vi "OCR Player Money ROI Only.vi"(7 "error in":errorcluster) -> (17 "String (Player10 Money)":string, 18 "String (Player 9 Money)":string, 19 "String (Player8 Money)":string, 20 "String (Player1 Money)":string, 21 "String (Player2 Money)":string, 22 "String (Player3 Money)":string, 23 "String (Player4 Money)":string, 24 "String (Player5 Money)":string, 25 "String (Player6 Money)":string, 26 "String (Player7 Money)":string, 27 "error out":errorcluster)   [LabVIEW 2015]
uses:
  <vilib>/vision/NI_Vision_Development_Module.lvlib
panel:
  out "appended array 2":T1(array[cluster])=[{"Global Rectangle"=[1068, 495, 1179, 512], "Contours"=[{"ID"=enum."External", "Type"=3, "Coordinates"=[1068, 495, 1179, 512]}]}, {"Global Rectangle"=[1068, 495, 1179, 512], "Contours"=[{"ID"=enum."External", "Type"=3, "Coordinates"=[1068, 495, 1179, 512]}]}, {"Global Rectangle"=[1385, 697, 1502, 712], "Contours"=[{"ID"=enum."External", "Type"=3, "Coordinates"=[1385, 697, 1502, 712]}]}, {"Global Rectangle"=[1264, 838, 1374, 853], "Contours"=[{"ID"=enum."External", "Type"=3, "Coordinates"=[1264, 838, 1374, 853]}]}, {"Global Rectangle"=[1029, 868, 1143, 884], "Contours"=[{"ID"=enum."External", "Type"=3, "Coordinates"=[1029, 868, 1143, 884]}]}, {"Global Rectangle"=[757, 870, 877, 885], "Contours"=[{"ID"=enum."External", "Type"=3, "Coordinates"=[757, 870, 877, 885]}]}, {"Global Rectangle"=[543, 836, 661, 852], "Contours"=[{"ID"=enum."External", "Type"=3, "Coordinates"=[543, 836, 661, 852]}]}, {"Global Rectangle"=[386, 689, 502, 706], "Contours"=[{"ID"=enum."External", "Type"=3, "Coordinates"=[386, 689, 502, 706]}]}, {"Global Rectangle"=[523, 533, 645, 550], "Contours"=[{"ID"=enum."External", "Type"=3, "Coordinates"=[523, 533, 645, 550]}]}, {"Global Rectangle"=[720, 494, 833, 510], "Contours"=[{"ID"=enum."External", "Type"=3, "Coordinates"=[720, 494, 833, 510]}]}]
  out "appended array":T1(array[cluster])
  out "Player Money":string[](array[string])
  in  "SS Path":path=path "c:/PokerSS/SS.png"
  out "Image Out":T2(plugin-control)
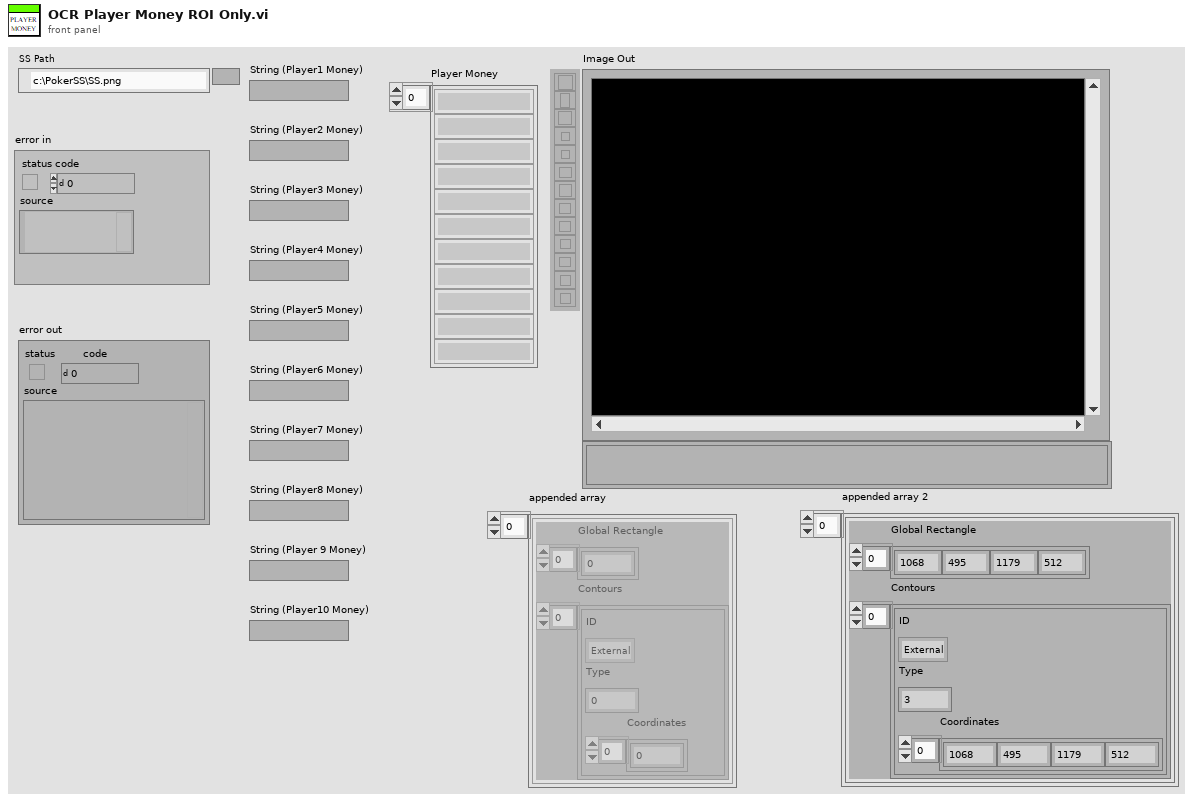
[diagram p1: front panel]
types:
  T1 = cluster{"Global Rectangle":i32[], "Contours":cluster{"ID":enum32{"External", "Internal"}, "Type":u32, "Coordinates":i32[]}[]}[]
  T2 = typedef "IMAQ Image.ctl" = refnum<image>
  T3 = cluster{"Threshold Data":cluster{"Method":enum16{"Fixed Range", "Uniform", "Linear", "Non Linear", "Local", "Color"}, "Looking for":u32, "Color Mode":u32, "Kernel Size":cluster{"Width":i32, "Height":i32}, "Ranges":cluster{"Min":i32, "Max":i32}[]}, "Reject Border":bool, "Number Of Erosions":i32, "Size & Spacing":cluster{"Segment Algorithm":u16, "Min Bounding Rect Width":i32, "Max Bounding Rect Width":i32, "Min Bounding Rect Height":i32, "Max Bounding Rect Height":i32, "Min Character Size":i32, "Max Character Size":i32, "Min Char Spacing":i32, "Max Horiz Element Spacing":i32, "Max Vert Element Spacing":i32, "Max Space Distance":i32}, "Read Options":cluster{"Read Strategy":i32, "Read Resolution":i32, "Scale Dependant":bool, "Aspect Ratio":i32, "Acceptance Level":i32, "Substitution Character":string, "MultiLine":bool}, "Valid Characters":cluster{"Pre-defined characters":i32, "User-defined characters":string}[], "Use Text Pattern":bool, "Orientation":u32, "# Lines Expected":u32, "Number of Blocks":i32}
  T4 = cluster{"Global Rectangle":i32[], "Contours":cluster{"ID":enum32{"External", "Internal"}, "Type":u32, "Coordinates":i32[]}[]}
  T5 = typedef "Image Type" = u32
  T6 = typedef "IMAQ OCR Session.ctl" = refnum<k1>
diagram:
  (unwired) path "C:/Users/Bob Dabalina/Documents/Labview/OCR Practice/Views Numbers.abc" ("File Path")
  w47 = u32 0 items=["Grayscale", "Binary", "Gradient", "Rainbow", "Temperature", "User Defined", "Binary 16 Bit", "Gradient 16 Bit", "Rainbow 16 Bit", "Temperature 16 Bit", "User Defined 16 Bit"] ("Palette Type")
  w56 = T3 {"Threshold Data"={"Method"=enum."Uniform", "Looking for"=1, "Color Mode"=0, "Kernel Size"={"Width"=32, "Height"=32}, "Ranges"=[{"Min"=1, "Max"=255}]}, "Reject Border"=TRUE, "Number Of Erosions"=0, "Size & Spacing"={"Segment Algorithm"=0, "Min Bounding Rect Width"=2, "Max Bounding Rect Width"=8, "Min Bounding Rect Height"=2, "Max Bounding Rect Height"=65536, "Min Character Size"=4, "Max Character Size"=5555, "Min Char Spacing"=1, "Max Horiz Element Spacing"=1, "Max Vert Element Spacing"=0, "Max Space Distance"=65536}, "Read Options"={"Read Strategy"=1, "Read Resolution"=2, "Scale Dependant"=FALSE, "Aspect Ratio"=400, "Acceptance Level"=700, "Substitution Character"="?", "MultiLine"=FALSE}, "Valid Characters"=[], "Use Text Pattern"=FALSE, "Orientation"=0, "# Lines Expected"=0, "Number of Blocks"=4}  # Parameters
  w2 = T4 {"Global Rectangle"=[720, 494, 833, 510], "Contours"=[{"ID"=enum."External", "Type"=3, "Coordinates"=[720, 494, 833, 510]}]}  # ROI Descriptor
  w64 = T3 {"Threshold Data"={"Method"=enum."Uniform", "Looking for"=1, "Color Mode"=0, "Kernel Size"={"Width"=32, "Height"=32}, "Ranges"=[{"Min"=1, "Max"=255}]}, "Reject Border"=TRUE, "Number Of Erosions"=0, "Size & Spacing"={"Segment Algorithm"=0, "Min Bounding Rect Width"=2, "Max Bounding Rect Width"=8, "Min Bounding Rect Height"=2, "Max Bounding Rect Height"=65536, "Min Character Size"=4, "Max Character Size"=5555, "Min Char Spacing"=1, "Max Horiz Element Spacing"=1, "Max Vert Element Spacing"=0, "Max Space Distance"=65536}, "Read Options"={"Read Strategy"=1, "Read Resolution"=2, "Scale Dependant"=FALSE, "Aspect Ratio"=400, "Acceptance Level"=700, "Substitution Character"="?", "MultiLine"=FALSE}, "Valid Characters"=[], "Use Text Pattern"=FALSE, "Orientation"=0, "# Lines Expected"=0, "Number of Blocks"=4}  # Parameters
  w4 = T4 {"Global Rectangle"=[523, 533, 645, 550], "Contours"=[{"ID"=enum."External", "Type"=3, "Coordinates"=[523, 533, 645, 550]}]}  # ROI Descriptor
  w72 = T3 {"Threshold Data"={"Method"=enum."Uniform", "Looking for"=1, "Color Mode"=0, "Kernel Size"={"Width"=32, "Height"=32}, "Ranges"=[{"Min"=1, "Max"=255}]}, "Reject Border"=TRUE, "Number Of Erosions"=0, "Size & Spacing"={"Segment Algorithm"=0, "Min Bounding Rect Width"=2, "Max Bounding Rect Width"=8, "Min Bounding Rect Height"=2, "Max Bounding Rect Height"=65536, "Min Character Size"=4, "Max Character Size"=5555, "Min Char Spacing"=1, "Max Horiz Element Spacing"=1, "Max Vert Element Spacing"=0, "Max Space Distance"=65536}, "Read Options"={"Read Strategy"=1, "Read Resolution"=2, "Scale Dependant"=FALSE, "Aspect Ratio"=400, "Acceptance Level"=700, "Substitution Character"="?", "MultiLine"=FALSE}, "Valid Characters"=[], "Use Text Pattern"=FALSE, "Orientation"=0, "# Lines Expected"=0, "Number of Blocks"=4}  # Parameters
  w6 = T4 {"Global Rectangle"=[386, 689, 502, 706], "Contours"=[{"ID"=enum."External", "Type"=3, "Coordinates"=[386, 689, 502, 706]}]}  # ROI Descriptor
  w80 = T3 {"Threshold Data"={"Method"=enum."Uniform", "Looking for"=1, "Color Mode"=0, "Kernel Size"={"Width"=32, "Height"=32}, "Ranges"=[{"Min"=1, "Max"=255}]}, "Reject Border"=TRUE, "Number Of Erosions"=0, "Size & Spacing"={"Segment Algorithm"=0, "Min Bounding Rect Width"=2, "Max Bounding Rect Width"=8, "Min Bounding Rect Height"=2, "Max Bounding Rect Height"=65536, "Min Character Size"=4, "Max Character Size"=5555, "Min Char Spacing"=1, "Max Horiz Element Spacing"=1, "Max Vert Element Spacing"=0, "Max Space Distance"=65536}, "Read Options"={"Read Strategy"=1, "Read Resolution"=2, "Scale Dependant"=FALSE, "Aspect Ratio"=400, "Acceptance Level"=700, "Substitution Character"="?", "MultiLine"=FALSE}, "Valid Characters"=[], "Use Text Pattern"=FALSE, "Orientation"=0, "# Lines Expected"=0, "Number of Blocks"=4}  # Parameters
  w8 = T4 {"Global Rectangle"=[543, 836, 661, 852], "Contours"=[{"ID"=enum."External", "Type"=3, "Coordinates"=[543, 836, 661, 852]}]}  # ROI Descriptor
  w88 = T3 {"Threshold Data"={"Method"=enum."Uniform", "Looking for"=1, "Color Mode"=0, "Kernel Size"={"Width"=32, "Height"=32}, "Ranges"=[{"Min"=1, "Max"=255}]}, "Reject Border"=TRUE, "Number Of Erosions"=0, "Size & Spacing"={"Segment Algorithm"=0, "Min Bounding Rect Width"=2, "Max Bounding Rect Width"=8, "Min Bounding Rect Height"=2, "Max Bounding Rect Height"=65536, "Min Character Size"=4, "Max Character Size"=5555, "Min Char Spacing"=1, "Max Horiz Element Spacing"=1, "Max Vert Element Spacing"=0, "Max Space Distance"=65536}, "Read Options"={"Read Strategy"=1, "Read Resolution"=2, "Scale Dependant"=FALSE, "Aspect Ratio"=400, "Acceptance Level"=700, "Substitution Character"="?", "MultiLine"=FALSE}, "Valid Characters"=[], "Use Text Pattern"=FALSE, "Orientation"=0, "# Lines Expected"=0, "Number of Blocks"=4}  # Parameters
  w10 = T4 {"Global Rectangle"=[757, 870, 877, 885], "Contours"=[{"ID"=enum."External", "Type"=3, "Coordinates"=[757, 870, 877, 885]}]}  # ROI Descriptor
  w96 = T3 {"Threshold Data"={"Method"=enum."Uniform", "Looking for"=1, "Color Mode"=0, "Kernel Size"={"Width"=32, "Height"=32}, "Ranges"=[{"Min"=1, "Max"=255}]}, "Reject Border"=TRUE, "Number Of Erosions"=0, "Size & Spacing"={"Segment Algorithm"=0, "Min Bounding Rect Width"=2, "Max Bounding Rect Width"=8, "Min Bounding Rect Height"=2, "Max Bounding Rect Height"=65536, "Min Character Size"=4, "Max Character Size"=5555, "Min Char Spacing"=1, "Max Horiz Element Spacing"=1, "Max Vert Element Spacing"=0, "Max Space Distance"=65536}, "Read Options"={"Read Strategy"=1, "Read Resolution"=2, "Scale Dependant"=FALSE, "Aspect Ratio"=400, "Acceptance Level"=700, "Substitution Character"="?", "MultiLine"=FALSE}, "Valid Characters"=[], "Use Text Pattern"=FALSE, "Orientation"=0, "# Lines Expected"=0, "Number of Blocks"=4}  # Parameters
  w12 = T4 {"Global Rectangle"=[1029, 868, 1143, 884], "Contours"=[{"ID"=enum."External", "Type"=3, "Coordinates"=[1029, 868, 1143, 884]}]}  # ROI Descriptor
  w104 = T3 {"Threshold Data"={"Method"=enum."Uniform", "Looking for"=1, "Color Mode"=0, "Kernel Size"={"Width"=32, "Height"=32}, "Ranges"=[{"Min"=1, "Max"=255}]}, "Reject Border"=TRUE, "Number Of Erosions"=0, "Size & Spacing"={"Segment Algorithm"=0, "Min Bounding Rect Width"=2, "Max Bounding Rect Width"=8, "Min Bounding Rect Height"=2, "Max Bounding Rect Height"=65536, "Min Character Size"=4, "Max Character Size"=5555, "Min Char Spacing"=1, "Max Horiz Element Spacing"=1, "Max Vert Element Spacing"=0, "Max Space Distance"=65536}, "Read Options"={"Read Strategy"=1, "Read Resolution"=2, "Scale Dependant"=FALSE, "Aspect Ratio"=400, "Acceptance Level"=700, "Substitution Character"="?", "MultiLine"=FALSE}, "Valid Characters"=[], "Use Text Pattern"=FALSE, "Orientation"=0, "# Lines Expected"=0, "Number of Blocks"=4}  # Parameters
  w14 = T4 {"Global Rectangle"=[1264, 838, 1374, 853], "Contours"=[{"ID"=enum."External", "Type"=3, "Coordinates"=[1264, 838, 1374, 853]}]}  # ROI Descriptor
  w112 = T3 {"Threshold Data"={"Method"=enum."Uniform", "Looking for"=1, "Color Mode"=0, "Kernel Size"={"Width"=32, "Height"=32}, "Ranges"=[{"Min"=1, "Max"=255}]}, "Reject Border"=TRUE, "Number Of Erosions"=0, "Size & Spacing"={"Segment Algorithm"=0, "Min Bounding Rect Width"=2, "Max Bounding Rect Width"=8, "Min Bounding Rect Height"=2, "Max Bounding Rect Height"=65536, "Min Character Size"=4, "Max Character Size"=5555, "Min Char Spacing"=1, "Max Horiz Element Spacing"=1, "Max Vert Element Spacing"=0, "Max Space Distance"=65536}, "Read Options"={"Read Strategy"=1, "Read Resolution"=2, "Scale Dependant"=FALSE, "Aspect Ratio"=400, "Acceptance Level"=700, "Substitution Character"="?", "MultiLine"=FALSE}, "Valid Characters"=[], "Use Text Pattern"=FALSE, "Orientation"=0, "# Lines Expected"=0, "Number of Blocks"=4}  # Parameters
  w16 = T4 {"Global Rectangle"=[1385, 697, 1502, 712], "Contours"=[{"ID"=enum."External", "Type"=3, "Coordinates"=[1385, 697, 1502, 712]}]}  # ROI Descriptor
  w120 = T3 {"Threshold Data"={"Method"=enum."Uniform", "Looking for"=1, "Color Mode"=0, "Kernel Size"={"Width"=32, "Height"=32}, "Ranges"=[{"Min"=1, "Max"=255}]}, "Reject Border"=TRUE, "Number Of Erosions"=0, "Size & Spacing"={"Segment Algorithm"=0, "Min Bounding Rect Width"=2, "Max Bounding Rect Width"=8, "Min Bounding Rect Height"=2, "Max Bounding Rect Height"=65536, "Min Character Size"=4, "Max Character Size"=5555, "Min Char Spacing"=1, "Max Horiz Element Spacing"=1, "Max Vert Element Spacing"=0, "Max Space Distance"=65536}, "Read Options"={"Read Strategy"=1, "Read Resolution"=2, "Scale Dependant"=FALSE, "Aspect Ratio"=400, "Acceptance Level"=700, "Substitution Character"="?", "MultiLine"=FALSE}, "Valid Characters"=[], "Use Text Pattern"=FALSE, "Orientation"=0, "# Lines Expected"=0, "Number of Blocks"=4}  # Parameters
  w18 = T4 {"Global Rectangle"=[1068, 495, 1179, 512], "Contours"=[{"ID"=enum."External", "Type"=3, "Coordinates"=[1068, 495, 1179, 512]}]}  # ROI Descriptor
  w128 = T3 {"Threshold Data"={"Method"=enum."Uniform", "Looking for"=1, "Color Mode"=0, "Kernel Size"={"Width"=32, "Height"=32}, "Ranges"=[{"Min"=1, "Max"=255}]}, "Reject Border"=TRUE, "Number Of Erosions"=0, "Size & Spacing"={"Segment Algorithm"=0, "Min Bounding Rect Width"=2, "Max Bounding Rect Width"=8, "Min Bounding Rect Height"=2, "Max Bounding Rect Height"=65536, "Min Character Size"=4, "Max Character Size"=5555, "Min Char Spacing"=1, "Max Horiz Element Spacing"=1, "Max Vert Element Spacing"=0, "Max Space Distance"=65536}, "Read Options"={"Read Strategy"=1, "Read Resolution"=2, "Scale Dependant"=FALSE, "Aspect Ratio"=400, "Acceptance Level"=700, "Substitution Character"="?", "MultiLine"=FALSE}, "Valid Characters"=[], "Use Text Pattern"=FALSE, "Orientation"=0, "# Lines Expected"=0, "Number of Blocks"=4}  # Parameters
  w21 = T4 {"Global Rectangle"=[1068, 495, 1179, 512], "Contours"=[{"ID"=enum."External", "Type"=3, "Coordinates"=[1068, 495, 1179, 512]}]}  # ROI Descriptor
  w131 = 1 items=["Red", "Green", "Blue", "Hue", "Saturation", "Luminance", "Value", "Intensity"] ("Color Plane")
  w132 = T5 4 items=["Grayscale (U8)", "Grayscale (I16)", "Grayscale (SGL)", "Complex (CSG)", "RGB (U32)", "HSL (U32)", "RGB (U64)", "Grayscale (U16)"] ("Image Type")
  # "Create player money array"
  n1 = Call Chain() -> (call chain=w134:string[])
  n2 = Index Array(array=w134) -> (element=w133:string)  [unwired: 1 in]
  n3 = call "IMAQ Create"("Image Name"=w133, "Image Type"=w132, "error in (no error)"="error in") -> ("New Image"=w137:T2, "error out"=w136:errorcluster)  [unwired: 1 in, 1 out]
  n4 = call "IMAQ ReadFile"("File Path"="SS Path", "error in (no error)"=w136, "Image"=w137) -> ("error out"=w138:errorcluster, "Image Out"=w130:T2)  [unwired: 2 in, 5 out]
  n5 = call "IMAQ ExtractSingleColorPlane"("Color Plane"=w131, "error in (no error)"=w138, "Image Src"=w130) -> ("error out"=w129:errorcluster, "Image Dst Out"=w48:T2)  [unwired: 1 in, 6 out]
  "Image Out" <- w48
  n6 = Initialize Array(w21, 1 ("dimension size")) -> (w19:T1)
  n7 = while "Create an OCR session and read the character set file.\nSet paramaters from Vision Assistant Step." {
    shift-right: [w143] -> w126
    shift-left: _ -> [w142]
    tunnel: w129 -> [w145]
    tunnel: w128 -> [w141]
    tunnel: path "C:/Users/Bob Dabalina/Documents/Labview/OCR Practice/Views Numbers.abc" ("File Path") -> [w140]
    tunnel: [w139] -> w127
    stop <- FALSE continue-if-true
    n8 = First Call?() -> (First Call?: T/F=w144:bool)
    n9 = case shown="True" w144 {
      tunnel: w140 -> [_ w152]
      tunnel: w145 -> [w147 w156]
      tunnel: [w148 w154] -> w143
      tunnel: [w147 w153] -> w139
      tunnel: w141 -> [_ w149]
      tunnel: w142 -> [w148 _]
      frame False {
      }
      frame True {
        w157 = 0 items=["Read All", "Read Character Set Only", "Read Properties Only"] ("Read Options")
        n10 = call <vilib>:"IVA Get Alternate Path.vi"("Path In"=w152) -> ("Path Out"=w151:path)  [unwired: 10 out]
        n11 = call "IMAQ OCR Create Session"("error in (no error)"=w156) -> ("error out"=w158:errorcluster, "IMAQ OCR Session"=w159:T6)  [unwired: 9 out]
        n12 = call "IMAQ OCR Read Character Set File"("File Path"=w151, "error in (no error)"=w158, "Read Options"=w157, "IMAQ OCR Session"=w159) -> ("error out"=w155:errorcluster, "IMAQ OCR Session (dup)"=w150:T6)  [unwired: 1 in, 5 out]
        n13 = call <vilib>:"IVA OCR - Set Parameters 2.vi"("error in (no error)"=w155, "Parameters"=w149, "IMAQ OCR Session"=w150) -> ("error out"=w153:errorcluster, "IMAQ OCR Session Out"=w154:T6)  [unwired: 7 in]
      }
    }
  }
  n14 = Unbundle By Name(w128) -> ("# Lines Expected"=w124:u32, "Orientation"=w125:u32)
  n15 = call "IMAQ OCR Read Text 4"("IMAQ OCR Session"=w126, "ROI Descriptor"=w21, "Image"=w48, "Number of Lines Requested"=w124, "error in (no error)"=w127, "Orientation"=w125) -> ("Read String"=w41:string, "error out"=w123:errorcluster)  [unwired: 8 out]
  "String (Player1 Money)" <- w41
  n16 = call <vilib>:"IVA Clear Coordsys Errors.vi"("error in (no error)"=w123) -> ("error out"=w122:errorcluster)  [unwired: 10 in]
  n17 = Initialize Array("") -> (w43:string[])  [unwired: 1 in]
  n18 = Insert Into Array(array=w43, index=0, new element=w41) -> (w40:string[])
  n19 = Build Array (concatenate)(w19, w18) -> (w17:T1)
  n20 = while "Create an OCR session and read the character set file.\nSet paramaters from Vision Assistant Step." {
    shift-right: [w164] -> w118
    shift-left: _ -> [w163]
    tunnel: w122 -> [w166]
    tunnel: w120 -> [w162]
    tunnel: path "C:/Users/Bob Dabalina/Documents/Labview/OCR Practice/Views Numbers.abc" ("File Path") -> [w161]
    tunnel: [w160] -> w119
    stop <- FALSE continue-if-true
    n21 = First Call?() -> (First Call?: T/F=w165:bool)
    n22 = case shown="True" w165 {
      tunnel: w161 -> [_ w173]
      tunnel: w166 -> [w168 w177]
      tunnel: [w169 w175] -> w164
      tunnel: [w168 w174] -> w160
      tunnel: w162 -> [_ w170]
      tunnel: w163 -> [w169 _]
      frame False {
      }
      frame True {
        w178 = 0 items=["Read All", "Read Character Set Only", "Read Properties Only"] ("Read Options")
        n23 = call <vilib>:"IVA Get Alternate Path.vi"("Path In"=w173) -> ("Path Out"=w172:path)  [unwired: 10 out]
        n24 = call "IMAQ OCR Create Session"("error in (no error)"=w177) -> ("error out"=w179:errorcluster, "IMAQ OCR Session"=w180:T6)  [unwired: 9 out]
        n25 = call "IMAQ OCR Read Character Set File"("File Path"=w172, "error in (no error)"=w179, "Read Options"=w178, "IMAQ OCR Session"=w180) -> ("error out"=w176:errorcluster, "IMAQ OCR Session (dup)"=w171:T6)  [unwired: 1 in, 5 out]
        n26 = call <vilib>:"IVA OCR - Set Parameters 2.vi"("error in (no error)"=w176, "Parameters"=w170, "IMAQ OCR Session"=w171) -> ("error out"=w174:errorcluster, "IMAQ OCR Session Out"=w175:T6)  [unwired: 7 in]
      }
    }
  }
  n27 = Unbundle By Name(w120) -> ("# Lines Expected"=w116:u32, "Orientation"=w117:u32)
  n28 = call "IMAQ OCR Read Text 4"("IMAQ OCR Session"=w118, "ROI Descriptor"=w18, "Image"=w48, "Number of Lines Requested"=w116, "error in (no error)"=w119, "Orientation"=w117) -> ("Read String"=w39:string, "error out"=w115:errorcluster)  [unwired: 8 out]
  "String (Player2 Money)" <- w39
  n29 = call <vilib>:"IVA Clear Coordsys Errors.vi"("error in (no error)"=w115) -> ("error out"=w114:errorcluster)  [unwired: 10 in]
  n30 = Build Array (concatenate)(w40, w39) -> (w38:string[])
  n31 = Build Array (concatenate)(w17, w16) -> (w15:T1)
  n32 = while "Create an OCR session and read the character set file.\nSet paramaters from Vision Assistant Step." {
    shift-right: [w185] -> w110
    shift-left: _ -> [w184]
    tunnel: w114 -> [w187]
    tunnel: w112 -> [w183]
    tunnel: path "C:/Users/Bob Dabalina/Documents/Labview/OCR Practice/Views Numbers.abc" ("File Path") -> [w182]
    tunnel: [w181] -> w111
    stop <- FALSE continue-if-true
    n33 = First Call?() -> (First Call?: T/F=w186:bool)
    n34 = case shown="True" w186 {
      tunnel: w182 -> [_ w194]
      tunnel: w187 -> [w189 w198]
      tunnel: [w190 w196] -> w185
      tunnel: [w189 w195] -> w181
      tunnel: w183 -> [_ w191]
      tunnel: w184 -> [w190 _]
      frame False {
      }
      frame True {
        w199 = 0 items=["Read All", "Read Character Set Only", "Read Properties Only"] ("Read Options")
        n35 = call <vilib>:"IVA Get Alternate Path.vi"("Path In"=w194) -> ("Path Out"=w193:path)  [unwired: 10 out]
        n36 = call "IMAQ OCR Create Session"("error in (no error)"=w198) -> ("error out"=w200:errorcluster, "IMAQ OCR Session"=w201:T6)  [unwired: 9 out]
        n37 = call "IMAQ OCR Read Character Set File"("File Path"=w193, "error in (no error)"=w200, "Read Options"=w199, "IMAQ OCR Session"=w201) -> ("error out"=w197:errorcluster, "IMAQ OCR Session (dup)"=w192:T6)  [unwired: 1 in, 5 out]
        n38 = call <vilib>:"IVA OCR - Set Parameters 2.vi"("error in (no error)"=w197, "Parameters"=w191, "IMAQ OCR Session"=w192) -> ("error out"=w195:errorcluster, "IMAQ OCR Session Out"=w196:T6)  [unwired: 7 in]
      }
    }
  }
  n39 = Unbundle By Name(w112) -> ("# Lines Expected"=w108:u32, "Orientation"=w109:u32)
  n40 = call "IMAQ OCR Read Text 4"("IMAQ OCR Session"=w110, "ROI Descriptor"=w16, "Image"=w48, "Number of Lines Requested"=w108, "error in (no error)"=w111, "Orientation"=w109) -> ("Read String"=w37:string, "error out"=w107:errorcluster)  [unwired: 8 out]
  "String (Player3 Money)" <- w37
  n41 = call <vilib>:"IVA Clear Coordsys Errors.vi"("error in (no error)"=w107) -> ("error out"=w106:errorcluster)  [unwired: 10 in]
  n42 = Build Array (concatenate)(w38, w37) -> (w36:string[])
  n43 = Build Array (concatenate)(w15, w14) -> (w13:T1)
  n44 = while "Create an OCR session and read the character set file.\nSet paramaters from Vision Assistant Step." {
    shift-right: [w206] -> w102
    shift-left: _ -> [w205]
    tunnel: w106 -> [w208]
    tunnel: w104 -> [w204]
    tunnel: path "C:/Users/Bob Dabalina/Documents/Labview/OCR Practice/Views Numbers.abc" ("File Path") -> [w203]
    tunnel: [w202] -> w103
    stop <- FALSE continue-if-true
    n45 = First Call?() -> (First Call?: T/F=w207:bool)
    n46 = case shown="True" w207 {
      tunnel: w203 -> [_ w215]
      tunnel: w208 -> [w210 w219]
      tunnel: [w211 w217] -> w206
      tunnel: [w210 w216] -> w202
      tunnel: w204 -> [_ w212]
      tunnel: w205 -> [w211 _]
      frame False {
      }
      frame True {
        w220 = 0 items=["Read All", "Read Character Set Only", "Read Properties Only"] ("Read Options")
        n47 = call <vilib>:"IVA Get Alternate Path.vi"("Path In"=w215) -> ("Path Out"=w214:path)  [unwired: 10 out]
        n48 = call "IMAQ OCR Create Session"("error in (no error)"=w219) -> ("error out"=w221:errorcluster, "IMAQ OCR Session"=w222:T6)  [unwired: 9 out]
        n49 = call "IMAQ OCR Read Character Set File"("File Path"=w214, "error in (no error)"=w221, "Read Options"=w220, "IMAQ OCR Session"=w222) -> ("error out"=w218:errorcluster, "IMAQ OCR Session (dup)"=w213:T6)  [unwired: 1 in, 5 out]
        n50 = call <vilib>:"IVA OCR - Set Parameters 2.vi"("error in (no error)"=w218, "Parameters"=w212, "IMAQ OCR Session"=w213) -> ("error out"=w216:errorcluster, "IMAQ OCR Session Out"=w217:T6)  [unwired: 7 in]
      }
    }
  }
  n51 = Unbundle By Name(w104) -> ("# Lines Expected"=w100:u32, "Orientation"=w101:u32)
  n52 = call "IMAQ OCR Read Text 4"("IMAQ OCR Session"=w102, "ROI Descriptor"=w14, "Image"=w48, "Number of Lines Requested"=w100, "error in (no error)"=w103, "Orientation"=w101) -> ("Read String"=w35:string, "error out"=w99:errorcluster)  [unwired: 8 out]
  "String (Player4 Money)" <- w35
  n53 = call <vilib>:"IVA Clear Coordsys Errors.vi"("error in (no error)"=w99) -> ("error out"=w98:errorcluster)  [unwired: 10 in]
  n54 = Build Array (concatenate)(w36, w35) -> (w34:string[])
  n55 = Build Array (concatenate)(w13, w12) -> (w11:T1)
  n56 = while "Create an OCR session and read the character set file.\nSet paramaters from Vision Assistant Step." {
    shift-right: [w227] -> w94
    shift-left: _ -> [w226]
    tunnel: w98 -> [w229]
    tunnel: w96 -> [w225]
    tunnel: path "C:/Users/Bob Dabalina/Documents/Labview/OCR Practice/Views Numbers.abc" ("File Path") -> [w224]
    tunnel: [w223] -> w95
    stop <- FALSE continue-if-true
    n57 = First Call?() -> (First Call?: T/F=w228:bool)
    n58 = case shown="True" w228 {
      tunnel: w224 -> [_ w236]
      tunnel: w229 -> [w231 w240]
      tunnel: [w232 w238] -> w227
      tunnel: [w231 w237] -> w223
      tunnel: w225 -> [_ w233]
      tunnel: w226 -> [w232 _]
      frame False {
      }
      frame True {
        w241 = 0 items=["Read All", "Read Character Set Only", "Read Properties Only"] ("Read Options")
        n59 = call <vilib>:"IVA Get Alternate Path.vi"("Path In"=w236) -> ("Path Out"=w235:path)  [unwired: 10 out]
        n60 = call "IMAQ OCR Create Session"("error in (no error)"=w240) -> ("error out"=w242:errorcluster, "IMAQ OCR Session"=w243:T6)  [unwired: 9 out]
        n61 = call "IMAQ OCR Read Character Set File"("File Path"=w235, "error in (no error)"=w242, "Read Options"=w241, "IMAQ OCR Session"=w243) -> ("error out"=w239:errorcluster, "IMAQ OCR Session (dup)"=w234:T6)  [unwired: 1 in, 5 out]
        n62 = call <vilib>:"IVA OCR - Set Parameters 2.vi"("error in (no error)"=w239, "Parameters"=w233, "IMAQ OCR Session"=w234) -> ("error out"=w237:errorcluster, "IMAQ OCR Session Out"=w238:T6)  [unwired: 7 in]
      }
    }
  }
  n63 = Unbundle By Name(w96) -> ("# Lines Expected"=w92:u32, "Orientation"=w93:u32)
  n64 = call "IMAQ OCR Read Text 4"("IMAQ OCR Session"=w94, "ROI Descriptor"=w12, "Image"=w48, "Number of Lines Requested"=w92, "error in (no error)"=w95, "Orientation"=w93) -> ("Read String"=w33:string, "error out"=w91:errorcluster)  [unwired: 8 out]
  "String (Player5 Money)" <- w33
  n65 = call <vilib>:"IVA Clear Coordsys Errors.vi"("error in (no error)"=w91) -> ("error out"=w90:errorcluster)  [unwired: 10 in]
  n66 = Build Array (concatenate)(w34, w33) -> (w32:string[])
  n67 = Build Array (concatenate)(w11, w10) -> (w9:T1)
  n68 = while "Create an OCR session and read the character set file.\nSet paramaters from Vision Assistant Step." {
    shift-right: [w248] -> w86
    shift-left: _ -> [w247]
    tunnel: w90 -> [w250]
    tunnel: w88 -> [w246]
    tunnel: path "C:/Users/Bob Dabalina/Documents/Labview/OCR Practice/Views Numbers.abc" ("File Path") -> [w245]
    tunnel: [w244] -> w87
    stop <- FALSE continue-if-true
    n69 = First Call?() -> (First Call?: T/F=w249:bool)
    n70 = case shown="True" w249 {
      tunnel: w245 -> [_ w257]
      tunnel: w250 -> [w252 w261]
      tunnel: [w253 w259] -> w248
      tunnel: [w252 w258] -> w244
      tunnel: w246 -> [_ w254]
      tunnel: w247 -> [w253 _]
      frame False {
      }
      frame True {
        w262 = 0 items=["Read All", "Read Character Set Only", "Read Properties Only"] ("Read Options")
        n71 = call <vilib>:"IVA Get Alternate Path.vi"("Path In"=w257) -> ("Path Out"=w256:path)  [unwired: 10 out]
        n72 = call "IMAQ OCR Create Session"("error in (no error)"=w261) -> ("error out"=w263:errorcluster, "IMAQ OCR Session"=w264:T6)  [unwired: 9 out]
        n73 = call "IMAQ OCR Read Character Set File"("File Path"=w256, "error in (no error)"=w263, "Read Options"=w262, "IMAQ OCR Session"=w264) -> ("error out"=w260:errorcluster, "IMAQ OCR Session (dup)"=w255:T6)  [unwired: 1 in, 5 out]
        n74 = call <vilib>:"IVA OCR - Set Parameters 2.vi"("error in (no error)"=w260, "Parameters"=w254, "IMAQ OCR Session"=w255) -> ("error out"=w258:errorcluster, "IMAQ OCR Session Out"=w259:T6)  [unwired: 7 in]
      }
    }
  }
  n75 = Unbundle By Name(w88) -> ("# Lines Expected"=w84:u32, "Orientation"=w85:u32)
  n76 = call "IMAQ OCR Read Text 4"("IMAQ OCR Session"=w86, "ROI Descriptor"=w10, "Image"=w48, "Number of Lines Requested"=w84, "error in (no error)"=w87, "Orientation"=w85) -> ("Read String"=w31:string, "error out"=w83:errorcluster)  [unwired: 8 out]
  "String (Player6 Money)" <- w31
  n77 = call <vilib>:"IVA Clear Coordsys Errors.vi"("error in (no error)"=w83) -> ("error out"=w82:errorcluster)  [unwired: 10 in]
  n78 = Build Array (concatenate)(w32, w31) -> (w30:string[])
  n79 = Build Array (concatenate)(w9, w8) -> (w7:T1)
  n80 = while "Create an OCR session and read the character set file.\nSet paramaters from Vision Assistant Step." {
    shift-right: [w269] -> w78
    shift-left: _ -> [w268]
    tunnel: w82 -> [w271]
    tunnel: w80 -> [w267]
    tunnel: path "C:/Users/Bob Dabalina/Documents/Labview/OCR Practice/Views Numbers.abc" ("File Path") -> [w266]
    tunnel: [w265] -> w79
    stop <- FALSE continue-if-true
    n81 = First Call?() -> (First Call?: T/F=w270:bool)
    n82 = case shown="True" w270 {
      tunnel: w266 -> [_ w278]
      tunnel: w271 -> [w273 w282]
      tunnel: [w274 w280] -> w269
      tunnel: [w273 w279] -> w265
      tunnel: w267 -> [_ w275]
      tunnel: w268 -> [w274 _]
      frame False {
      }
      frame True {
        w283 = 0 items=["Read All", "Read Character Set Only", "Read Properties Only"] ("Read Options")
        n83 = call <vilib>:"IVA Get Alternate Path.vi"("Path In"=w278) -> ("Path Out"=w277:path)  [unwired: 10 out]
        n84 = call "IMAQ OCR Create Session"("error in (no error)"=w282) -> ("error out"=w284:errorcluster, "IMAQ OCR Session"=w285:T6)  [unwired: 9 out]
        n85 = call "IMAQ OCR Read Character Set File"("File Path"=w277, "error in (no error)"=w284, "Read Options"=w283, "IMAQ OCR Session"=w285) -> ("error out"=w281:errorcluster, "IMAQ OCR Session (dup)"=w276:T6)  [unwired: 1 in, 5 out]
        n86 = call <vilib>:"IVA OCR - Set Parameters 2.vi"("error in (no error)"=w281, "Parameters"=w275, "IMAQ OCR Session"=w276) -> ("error out"=w279:errorcluster, "IMAQ OCR Session Out"=w280:T6)  [unwired: 7 in]
      }
    }
  }
  n87 = Unbundle By Name(w80) -> ("# Lines Expected"=w76:u32, "Orientation"=w77:u32)
  n88 = call "IMAQ OCR Read Text 4"("IMAQ OCR Session"=w78, "ROI Descriptor"=w8, "Image"=w48, "Number of Lines Requested"=w76, "error in (no error)"=w79, "Orientation"=w77) -> ("Read String"=w29:string, "error out"=w75:errorcluster)  [unwired: 8 out]
  "String (Player7 Money)" <- w29
  n89 = call <vilib>:"IVA Clear Coordsys Errors.vi"("error in (no error)"=w75) -> ("error out"=w74:errorcluster)  [unwired: 10 in]
  n90 = Build Array (concatenate)(w30, w29) -> (w28:string[])
  n91 = Build Array (concatenate)(w7, w6) -> (w5:T1)
  n92 = while "Create an OCR session and read the character set file.\nSet paramaters from Vision Assistant Step." {
    shift-right: [w290] -> w70
    shift-left: _ -> [w289]
    tunnel: w74 -> [w292]
    tunnel: w72 -> [w288]
    tunnel: path "C:/Users/Bob Dabalina/Documents/Labview/OCR Practice/Views Numbers.abc" ("File Path") -> [w287]
    tunnel: [w286] -> w71
    stop <- FALSE continue-if-true
    n93 = First Call?() -> (First Call?: T/F=w291:bool)
    n94 = case shown="True" w291 {
      tunnel: w287 -> [_ w299]
      tunnel: w292 -> [w294 w303]
      tunnel: [w295 w301] -> w290
      tunnel: [w294 w300] -> w286
      tunnel: w288 -> [_ w296]
      tunnel: w289 -> [w295 _]
      frame False {
      }
      frame True {
        w304 = 0 items=["Read All", "Read Character Set Only", "Read Properties Only"] ("Read Options")
        n95 = call <vilib>:"IVA Get Alternate Path.vi"("Path In"=w299) -> ("Path Out"=w298:path)  [unwired: 10 out]
        n96 = call "IMAQ OCR Create Session"("error in (no error)"=w303) -> ("error out"=w305:errorcluster, "IMAQ OCR Session"=w306:T6)  [unwired: 9 out]
        n97 = call "IMAQ OCR Read Character Set File"("File Path"=w298, "error in (no error)"=w305, "Read Options"=w304, "IMAQ OCR Session"=w306) -> ("error out"=w302:errorcluster, "IMAQ OCR Session (dup)"=w297:T6)  [unwired: 1 in, 5 out]
        n98 = call <vilib>:"IVA OCR - Set Parameters 2.vi"("error in (no error)"=w302, "Parameters"=w296, "IMAQ OCR Session"=w297) -> ("error out"=w300:errorcluster, "IMAQ OCR Session Out"=w301:T6)  [unwired: 7 in]
      }
    }
  }
  n99 = Unbundle By Name(w72) -> ("# Lines Expected"=w68:u32, "Orientation"=w69:u32)
  n100 = call "IMAQ OCR Read Text 4"("IMAQ OCR Session"=w70, "ROI Descriptor"=w6, "Image"=w48, "Number of Lines Requested"=w68, "error in (no error)"=w71, "Orientation"=w69) -> ("Read String"=w27:string, "error out"=w67:errorcluster)  [unwired: 8 out]
  "String (Player8 Money)" <- w27
  n101 = call <vilib>:"IVA Clear Coordsys Errors.vi"("error in (no error)"=w67) -> ("error out"=w66:errorcluster)  [unwired: 10 in]
  n102 = Build Array (concatenate)(w28, w27) -> (w26:string[])
  n103 = Build Array (concatenate)(w5, w4) -> (w3:T1)
  n104 = while "Create an OCR session and read the character set file.\nSet paramaters from Vision Assistant Step." {
    shift-right: [w311] -> w62
    shift-left: _ -> [w310]
    tunnel: w66 -> [w313]
    tunnel: w64 -> [w309]
    tunnel: path "C:/Users/Bob Dabalina/Documents/Labview/OCR Practice/Views Numbers.abc" ("File Path") -> [w308]
    tunnel: [w307] -> w63
    stop <- FALSE continue-if-true
    n105 = First Call?() -> (First Call?: T/F=w312:bool)
    n106 = case shown="True" w312 {
      tunnel: w308 -> [_ w320]
      tunnel: w313 -> [w315 w324]
      tunnel: [w316 w322] -> w311
      tunnel: [w315 w321] -> w307
      tunnel: w309 -> [_ w317]
      tunnel: w310 -> [w316 _]
      frame False {
      }
      frame True {
        w325 = 0 items=["Read All", "Read Character Set Only", "Read Properties Only"] ("Read Options")
        n107 = call <vilib>:"IVA Get Alternate Path.vi"("Path In"=w320) -> ("Path Out"=w319:path)  [unwired: 10 out]
        n108 = call "IMAQ OCR Create Session"("error in (no error)"=w324) -> ("error out"=w326:errorcluster, "IMAQ OCR Session"=w327:T6)  [unwired: 9 out]
        n109 = call "IMAQ OCR Read Character Set File"("File Path"=w319, "error in (no error)"=w326, "Read Options"=w325, "IMAQ OCR Session"=w327) -> ("error out"=w323:errorcluster, "IMAQ OCR Session (dup)"=w318:T6)  [unwired: 1 in, 5 out]
        n110 = call <vilib>:"IVA OCR - Set Parameters 2.vi"("error in (no error)"=w323, "Parameters"=w317, "IMAQ OCR Session"=w318) -> ("error out"=w321:errorcluster, "IMAQ OCR Session Out"=w322:T6)  [unwired: 7 in]
      }
    }
  }
  n111 = Unbundle By Name(w64) -> ("# Lines Expected"=w60:u32, "Orientation"=w61:u32)
  n112 = call "IMAQ OCR Read Text 4"("IMAQ OCR Session"=w62, "ROI Descriptor"=w4, "Image"=w48, "Number of Lines Requested"=w60, "error in (no error)"=w63, "Orientation"=w61) -> ("Read String"=w25:string, "error out"=w59:errorcluster)  [unwired: 8 out]
  "String (Player 9 Money)" <- w25
  n113 = call <vilib>:"IVA Clear Coordsys Errors.vi"("error in (no error)"=w59) -> ("error out"=w58:errorcluster)  [unwired: 10 in]
  n114 = Build Array (concatenate)(w26, w25) -> (w24:string[])
  n115 = Build Array (concatenate)(w3, w2) -> (→"appended array":T1)
  n116 = while "Create an OCR session and read the character set file.\nSet paramaters from Vision Assistant Step." {
    shift-right: [w332] -> w54
    shift-left: _ -> [w331]
    tunnel: w58 -> [w334]
    tunnel: w56 -> [w330]
    tunnel: path "C:/Users/Bob Dabalina/Documents/Labview/OCR Practice/Views Numbers.abc" ("File Path") -> [w329]
    tunnel: [w328] -> w55
    stop <- FALSE continue-if-true
    n117 = First Call?() -> (First Call?: T/F=w333:bool)
    n118 = case shown="True" w333 {
      tunnel: w329 -> [_ w341]
      tunnel: w334 -> [w336 w345]
      tunnel: [w337 w343] -> w332
      tunnel: [w336 w342] -> w328
      tunnel: w330 -> [_ w338]
      tunnel: w331 -> [w337 _]
      frame False {
      }
      frame True {
        w346 = 0 items=["Read All", "Read Character Set Only", "Read Properties Only"] ("Read Options")
        n119 = call <vilib>:"IVA Get Alternate Path.vi"("Path In"=w341) -> ("Path Out"=w340:path)  [unwired: 10 out]
        n120 = call "IMAQ OCR Create Session"("error in (no error)"=w345) -> ("error out"=w347:errorcluster, "IMAQ OCR Session"=w348:T6)  [unwired: 9 out]
        n121 = call "IMAQ OCR Read Character Set File"("File Path"=w340, "error in (no error)"=w347, "Read Options"=w346, "IMAQ OCR Session"=w348) -> ("error out"=w344:errorcluster, "IMAQ OCR Session (dup)"=w339:T6)  [unwired: 1 in, 5 out]
        n122 = call <vilib>:"IVA OCR - Set Parameters 2.vi"("error in (no error)"=w344, "Parameters"=w338, "IMAQ OCR Session"=w339) -> ("error out"=w342:errorcluster, "IMAQ OCR Session Out"=w343:T6)  [unwired: 7 in]
      }
    }
  }
  n123 = Unbundle By Name(w56) -> ("# Lines Expected"=w52:u32, "Orientation"=w53:u32)
  n124 = call "IMAQ OCR Read Text 4"("IMAQ OCR Session"=w54, "ROI Descriptor"=w2, "Image"=w48, "Number of Lines Requested"=w52, "error in (no error)"=w55, "Orientation"=w53) -> ("Read String"=w23:string, "error out"=w51:errorcluster)  [unwired: 8 out]
  "String (Player10 Money)" <- w23
  n125 = call <vilib>:"IVA Clear Coordsys Errors.vi"("error in (no error)"=w51) -> ("error out"=w50:errorcluster)  [unwired: 10 in]
  n126 = property on="Image Out" class="ImageControl"(error in=w50, "Palette:Palette Type"=w47) -> (error out=→"error out":errorcluster)  [unwired: 1 in, 1 out]
  n127 = Build Array (concatenate)(w24, w23) -> (→"Player Money":string[])
